vi "IOCtrl_setT0.vi"(8 "error in (no error)":errorcluster) -> (0 "error out":errorcluster)   [LabVIEW 2015, in "ESLSCDLL.lvlib"]
uses:
  ESLSCDLL.lvlib
  Globals.vi
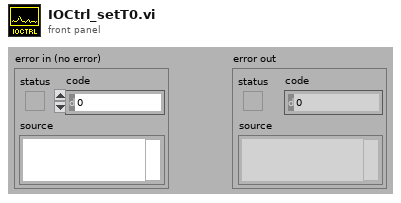
[diagram p1: front panel]
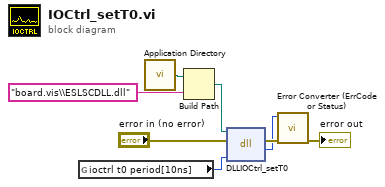
[diagram p0: block diagram]
diagram:
  n1 = global read "Globals.vi" "ioctrl t0 period[10ns]"() -> (w4:u32)
  n2 = call <vilib>:"Application Directory.vi"() -> ("Application Directory"=w3:path)
  n3 = Build Path(base path=w3, name or relative path="board.vis\\ESLSCDLL.dll") -> (appended path=w1:path)
  n4 = dll-call lib="C:/ENTW/PCIE/LV64/board.vis/ESLSCDLL.dll" fn="DLLIOCtrl_setT0" ("lwlscdll.dll:DLLSetTemp")(path in=w1, error in="error in (no error)", "period_in_10ns"=w4) -> (error out=w7:errorcluster, "es_status_codes"=w5:i32)  [unwired: 2 in, 1 out]
  n5 = call "Error Converter (ErrCode or Status).vi"("error in (no error)"=w7, "error code"=w5) -> ("error out"=→"error out":errorcluster)  [unwired: 9 in]
